vi "AudioTest.Pololu.Dual_Servo_Controller.vi"(11 "Module Config":T3={"Name"="DualServoCtrl", "Parent Q"=refnum, "Is Child?"=FALSE, "Index"=0, "Dirs"={"Root"=path "", "Config"=path "C:/ATE/Config", "Logs"=path "C:/ATE/Logs", "Reports"=path "C:/ATE/Reports", "App Data"=path "C:/ProgramData/MAIN"}, "Simulate"=FALSE, "SimCtrl"=refnum}) -> ()   [LabVIEW 2018]
uses:
  <vilib>/KATE/Module/Module Config.ctl
  <vilib>/KATE/Queues/Q.Element.ctl
  <vilib>/KATE/Module/Module.Working Dirs.ctl
  Common/Instruments/Servo Motors/Pololu/SubVIs/Pololu.Device Config.ctl
  Common/Instruments/Servo Motors/Pololu/SubVIs/Pololu.Device Range Config.ctl
  <vilib>/KATE/Module/Module.SW Version Info.ctl
  <vilib>/KATE/Module/Window/Window.Task, Action.ctl
  Common/Instruments/Servo Motors/Pololu/Dual Servo Manager Class/PololuCtrl.lvclass
  Common/Instruments/Servo Motors/Pololu/SubVIs/Pololu.Commands.ctl
  <vilib>/KATE/Config/Stored Controls/Class.SaveCtrls.lvclass
  <vilib>/KATE/Queues/Queue Utils.lvlib
  <vilib>/KATE/Module/Module Utils.lvlib
  <vilib>/KATE/Scheduler/Scheduler.lvlib
  <vilib>/KATE/Files/File Utils.lvlib
  <vilib>/KATE/Status/Status Utils.lvlib
  <vilib>/KATE/Event Log/Event Log.lvlib
panel:
  out "R Pos 3":dbl caption="Pos 0" format="%.1f"
  out "R Pos 2":dbl caption="Pos 1" format="%.1f"
  in  "Main Tab":enum32{"Operate", "Maint"}(tab)
  in  "Operate Tab":enum32{"Operate", "Config"}(tab)
  in  "Move All to 3":bool
  in  "R Step Dwn":bool
  in  "R Step Up":bool
  in  "L Step Dwn":bool
  in  "L Step Up":bool
  in  "Move All to 0":bool
  in  "Move All to 1":bool
  in  "R Go To Pos 0":bool
  in  "R Go To Pos 1":bool
  in  "Right Cmd Pos (Deg)":dbl(slide)=135.0 caption="Position (Deg)" max=270.0 scale=0.0..270.0 scale format="%.1f"
  out "R Pos 0":dbl caption="Pos 0" format="%.1f"
  out "R Pos 1":dbl caption="Pos 1" format="%.1f"
  in  "R Set Pos 0":bool
  in  "R Set Pos 1":bool
  in  "L Go To Pos 0":bool
  in  "L Go To Pos 1":bool
  in  "WaitTillDone":bool=TRUE caption="Wait Till Done"
  in  "Mov Timeout":dbl=5.0 caption="Timeout(s)"
  in  "Mov PosID":u8 caption="Position ID"
  in  "Mov Device":enum16{"Left", "Right", "All"}(ring)=enum."All" caption="Device"
  in  "Move Funct":bool
  in  "Left Cmd Pos (Deg)":dbl(slide)=135.0 caption="Position (Deg)" max=270.0 scale=0.0..270.0 scale format="%.1f"
  in  "Pos0 Invert":bool caption="Invert Scale"
  out "L Pos 0":dbl caption="Pos 0" format="%.1f"
  out "L Pos1":dbl caption="Pos 1" format="%.1f"
  in  "L Set Pos 0":bool
  in  "L Set Pos 1":bool
  out "Moving":bool
  in  "Pos1 Invert":bool caption="Invert Scale"
  out "Pos Cmd us":dbl[](array[numeric]) caption="Position Commands in us" format="%.1f"
  in  "0.25us/10ms/80ms":dbl=6.0
  in  "0.25us/10ms":dbl=100.0
  in  "Set Accel":bool
  in  "Set Speed":bool
  out "Read Errors":u16 max=270 format="%016b"
  in  "Get Errors":bool
  out "Error":errorcluster
  in  "Get Pos":bool
  out "Status Pos(Deg)":dbl[](array[numeric]) format="%.1f"
  out "Left Cmd Pos(us)":dbl
  out "Right Cmd Pos(us)":dbl
  in  "PID":string="0089"
  in  "VID":string="1FFB"
  out "Device Config":T1[](array[typedef])
  out "Config Dir":path
  out "CLI Args":string[](array[string])
  out "Connected":bool
  in  "Connect":bool
  in  "Disconnect":bool
  out "Port":string
  out "Error Status":string
  in  "R Set Upper Stop":bool
  out "R Upper Stop":dbl format="%.1f"
  in  "L Set Upper Stop":bool
  out "L Upper Stop":dbl format="%.1f"
  in  "L Set Lower Stop":bool
  out "L Lower Stop":dbl format="%.1f"
  in  "R Set Lower Stop":bool
  out "R Lower Stop":dbl format="%.1f"
  in  "Ignore Stops":bool=TRUE
  in  "Reset Stops":bool
  # "Detailed Function"
  # "Dual Servo Controller"
  # "Summary Functions"
  # "LEFT"
  # "RIGHT"
  # "Move(1,All)"
  # "Move(0,All)"
  # "Move(3,All)"
  # "Move(PosID,[Devices, Wait,Timeout])"
  # "Baby Step"
  # "Baby Step"
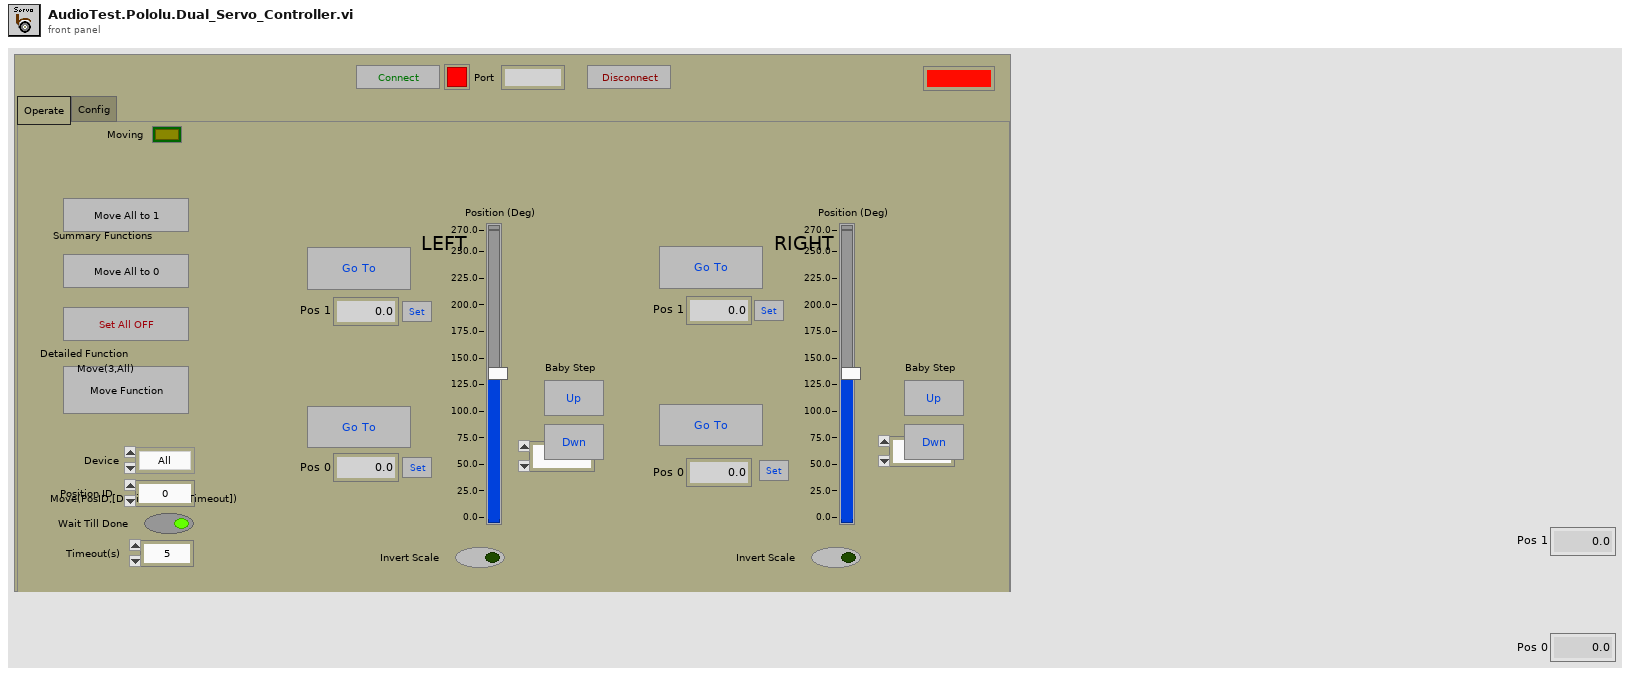
[diagram p1: front panel]
types:
  T1 = typedef "Pololu.Device Config.ctl" = cluster{"Chan":u8, "Accel":u16, "Speed":u16, "Positions":dbl[], "Range Info":T2}
  T2 = typedef "Pololu.Device Range Config.ctl" = cluster{"Min us":dbl, "Max us":dbl, "Min deg":dbl, "Max deg":dbl, "LStopDeg":dbl, "UStopDeg":dbl}
  T3 = typedef "KATE_Lib.lvlib/Module Utils.lvlib/Module Config.ctl" = cluster{"Name":string, "Parent Q":refnum<queue>, "Is Child?":bool, "Index":i32, "Dirs":T4, "Simulate":bool, "SimCtrl":refnum<vi>}
  T4 = typedef "KATE_Lib.lvlib/Module Utils.lvlib/Module.Working Dirs.ctl" = cluster{"Root":path, "Config":path, "Logs":path, "Reports":path, "App Data":path}
  T5 = typedef "KATE_Lib.lvlib/Module Utils.lvlib/Module.SW Version Info.ctl" = cluster{"AppName":string, "Company":string, "Version":string, "Description":string, "PN":string}
  T6 = typedef "KATE_Lib.lvlib/Module Utils.lvlib/Module Sys Info.ctl" = cluster{"Main Q":refnum<queue>, "Exe":bool, "SW Rev":T5, "Self Ref":refnum<vi>, "Main Tab":refnum<vi>, "Pane":refnum<vi>, "Stop":cluster{"Ref":refnum<event-registration>, "Event":refnum<user-event>}, "Cfg":T3, "Services":cluster{"Name":string, "vi ref":refnum<vi>}[], "Menu Ref":refnum<k9>, "CtrlStates":refnum<class "Class.SaveCtrls.lvclass">, "Docs":cluster{"Tags":string[], "Paths":path[]}, "Log":refnum<class "Event Notification.lvclass">, "Test Controls":refnum<vi>[], "Child Modules":cluster{"Name":string, "vi ref":refnum<vi>}[], "SW Items":string[][], "AppData":refnum<class "Class.AppData.lvclass">, "Subscriptions":refnum<class "Subscription.lvclass">}
  T7 = enum32{"Invalid", "Standard", "Closed", "Hidden", "Minimized", "Maximized"}
  T8 = enum16{"Left Upper Stop", "Left Lower Stop", "Left Pos 0", "Left Pos 1", "Right Upper Stop", "Right Lower Stop", "Right Pos 0", "Right Pos 1"}
  T9 = typedef "Pololu.Commands.ctl" = enum16{"Set Pos", "Set Speed", "Set Accel", "Get Pos", "Get Mov Status", "Get Errors"}
  T10 = cluster{"Active":bool, "Test":string, "Args":string[]}
  T11 = cluster{"Pololu":refnum<class "PololuCtrl.lvclass">, "CLI":cluster{"Active":bool, "Test":string, "Args":string[]}}
  T12 = cluster{"Device":enum16{"Left", "Right", "All"}, "PosID":u8, "Wait":bool, "Timeout":dbl}
  T13 = typedef "KATE_Lib.lvlib/Module Utils.lvlib/Window.Task, Action.ctl" = enum16{"Resize()", "Show Panel(Bool)", "Show Scroll Bars(Bool)", "Dock to SubPanel(SubPanel Ref)", "Undock from SubPanel()", "Return to SubPanel()", "Go To Maint Tab()", "Show Maint Tab(Bool)", "Open Block Diagram()"}
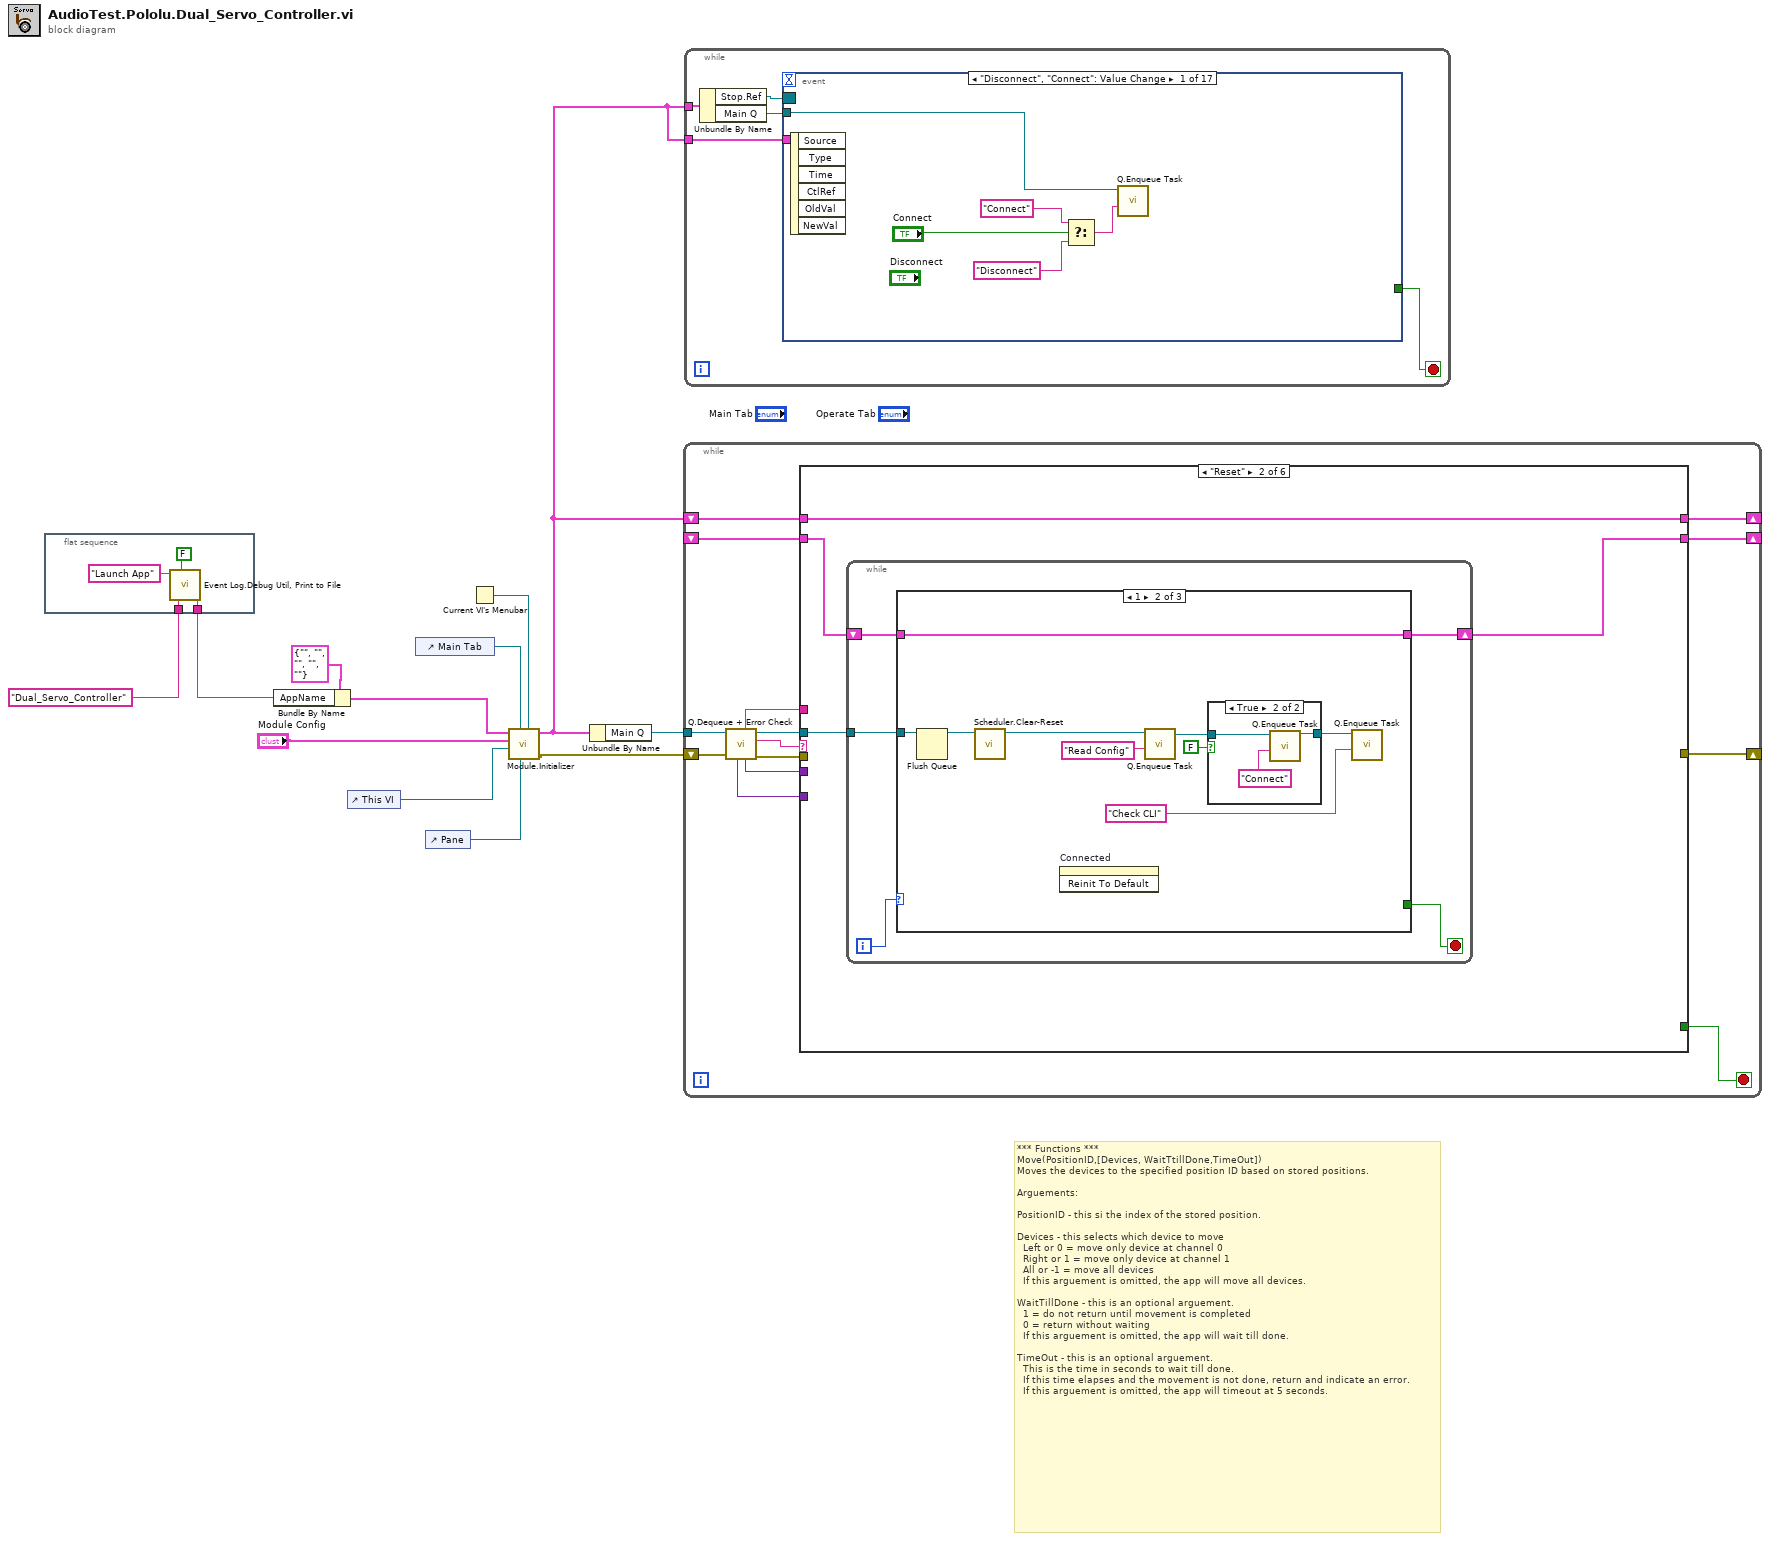
[diagram p0: block diagram]
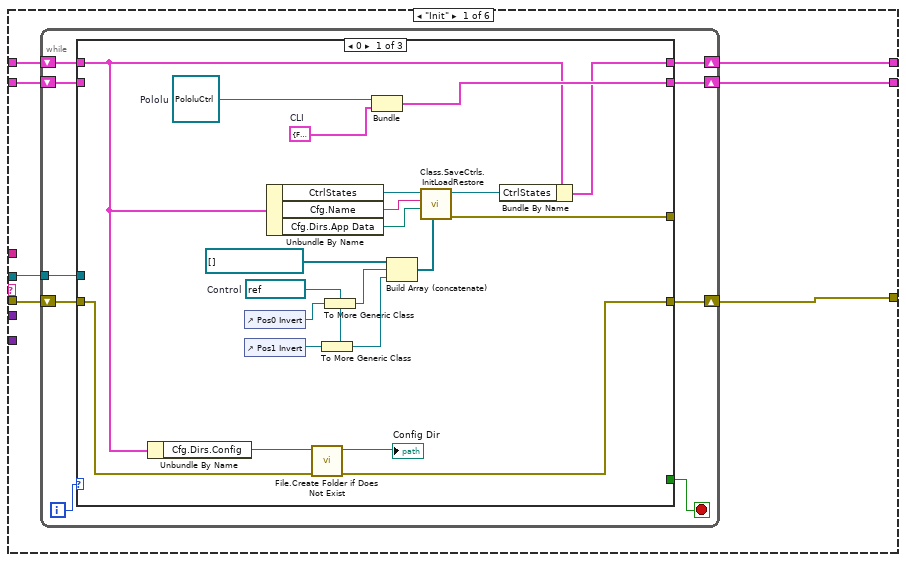
[diagram p2: hidden frame]
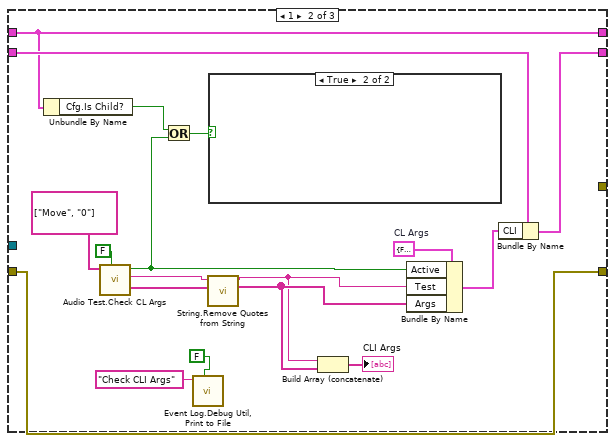
[diagram p3: hidden frame]
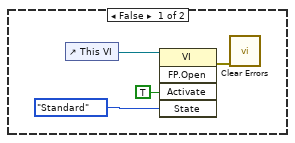
[diagram p4: hidden frame]
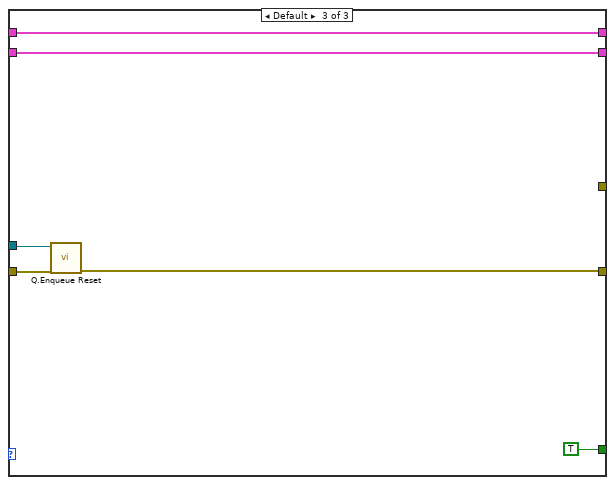
[diagram p5: hidden frame]
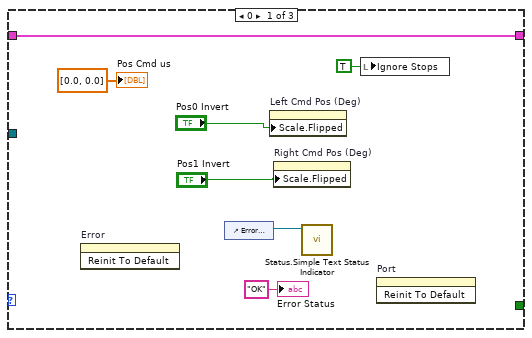
[diagram p6: hidden frame]
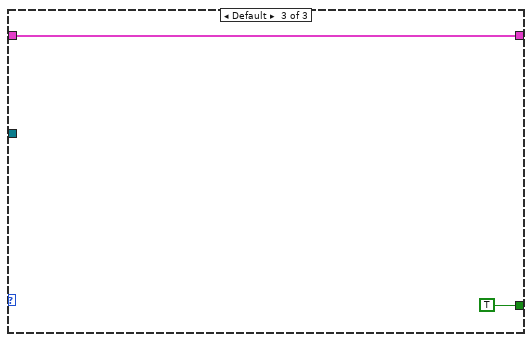
[diagram p8: hidden frame]
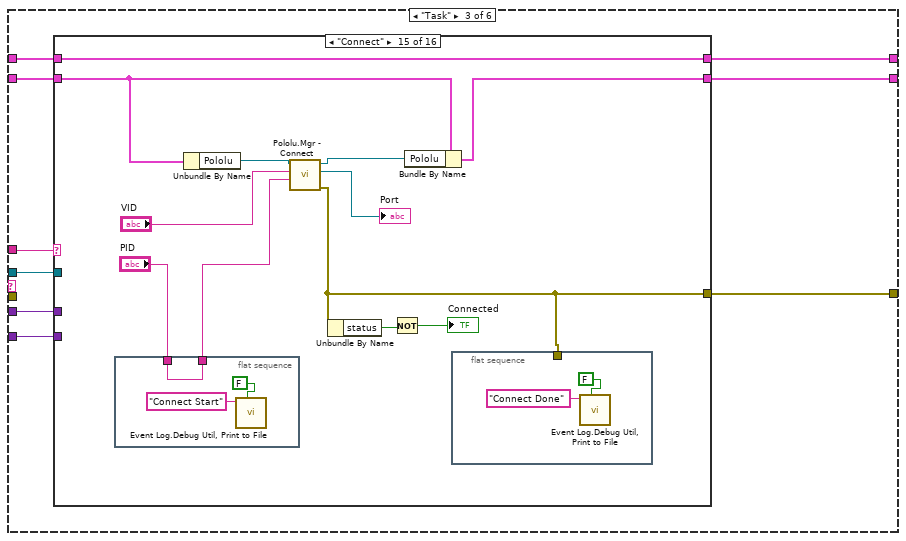
[diagram p9: hidden frame]
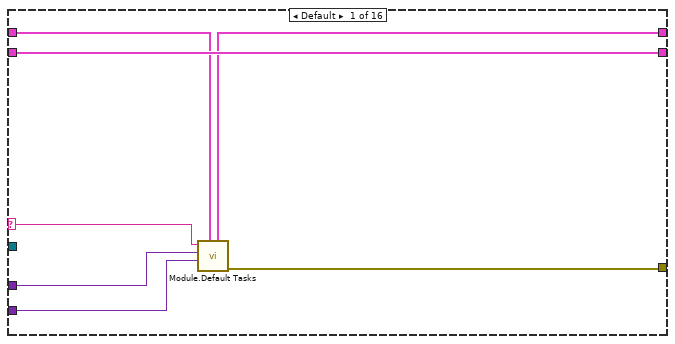
[diagram p10: hidden frame]
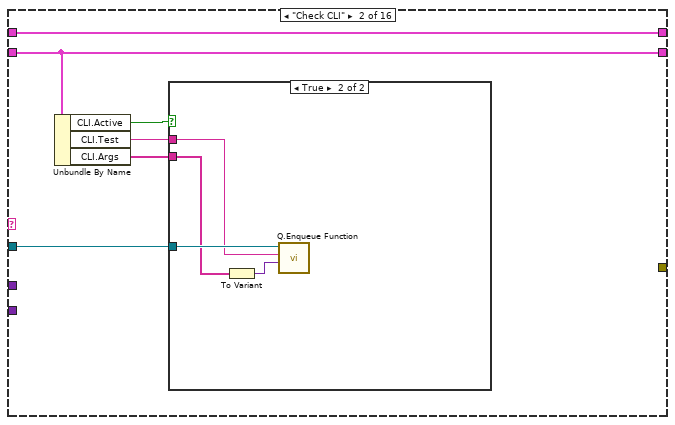
[diagram p11: hidden frame]
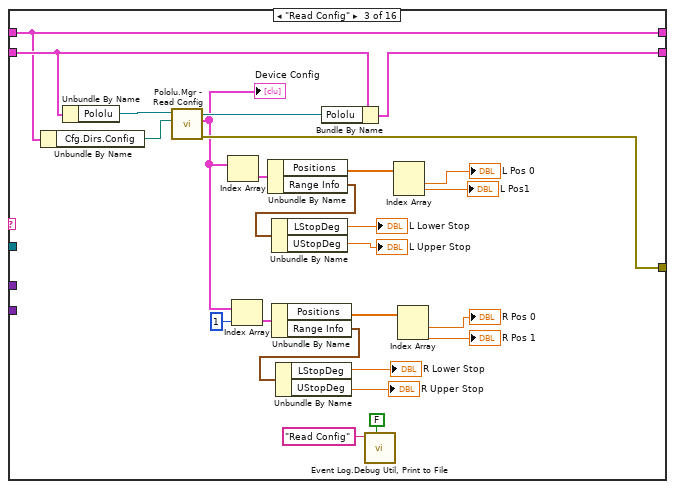
[diagram p13: hidden frame]
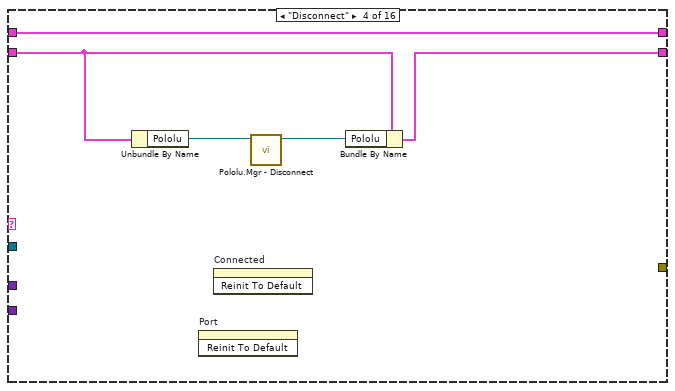
[diagram p14: hidden frame]
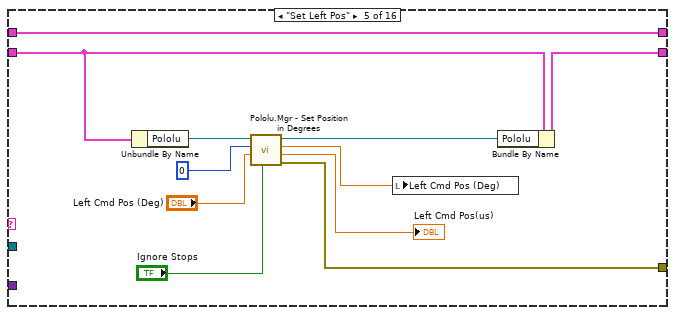
[diagram p15: hidden frame]
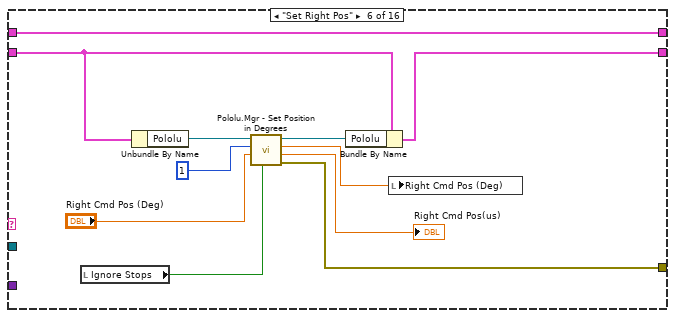
[diagram p16: hidden frame]
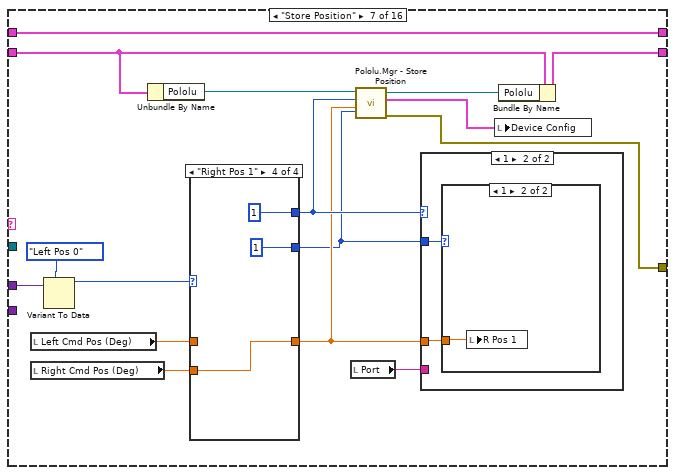
[diagram p17: hidden frame]
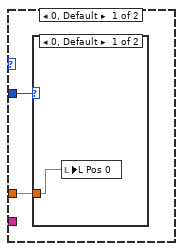
[diagram p18: hidden frame]
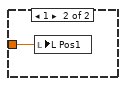
[diagram p19: hidden frame]
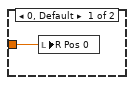
[diagram p20: hidden frame]
diagram:
  # "*** Functions ***\nMove(PositionID,[Devices, WaitTtillDone,TimeOut])\nMoves the devices to the specified position ID based on stored positions.\n\nArguements:\n\nPositionID - this si the index of the stored position.\n\nDevices - this selects which device to move\n  Left or 0 = move only device at channel 0\n  Right or 1 = move only device at channel 1\n  All or -1 = move all devices\n  If this arguement is omitted, the app will move all devices.\n\nWaitTillDone - this is an optional arguement.\n  1 = do not return until movement is completed\n  0 = return without waiting\n  If this arguement is omitted, the app will wait till done.\n\nTimeOut - this is an optional arguement.\n  This is the time in seconds to wait till done.\n  If this time elapses and the movement is not done, return and indicate an error.\n  If this arguement is omitted, the app will timeout at 5 seconds."
  n1 = flat-sequence {
    tunnel: [w14] -> w2
    tunnel: "Dual_Servo_Controller" ("AppName") -> [w14]
    frame #0 {
      n2 = call <vilib>:"Event Log.Debug Util, Print to File.vi"("Enable"=FALSE, "Message"="Launch App") -> ()  [unwired: 10 in]
    }
  }
  n3 = Bundle By Name(cluster=T5 {"AppName"="", "Company"="", "Version"="", "Description"="", "PN"=""} ("SW Rev"), "AppName"=w2) -> (w5:T5)
  n4 = control-ref of="This VI"() -> (w10:refnum<vi>)
  n5 = control-ref of="Main Tab"() -> (w8:refnum<vi>)
  n6 = control-ref of="Pane"() -> (w7:refnum<vi>)
  n7 = Current VI's Menubar() -> (w9:refnum<k9>)
  n8 = call <vilib>:"Module.Initializer.vi"("Menu Ref"=w9, "Pane"=w7, "Main Tab"=w8, "Self Ref"=w10, "Module Config"="Module Config", "SW Rev"=w5) -> ("error out"=w12:errorcluster, "Sys"=w3:T6)  [unwired: 4 in]
  n9 = Unbundle By Name(w3) -> ("Main Q"=w11:refnum<queue>)
  n10 = while {
    tunnel: w11 -> [w29]
    shift-right: [w20] -> _
    shift-left: w12 -> [w28]
    shift-right: [w18] -> _
    shift-left: _ -> [w22]
    shift-right: [w16] -> _
    shift-left: w3 -> [w17]
    stop <- w19 stop-if-true
    n11 = call <vilib>:"Q.Dequeue + Error Check.vi"("Error In"=w28, "Q In"=w29) -> ("error out"=w21:errorcluster, "Cmd"=w27:string, "Q Out"=w26:refnum<queue>, "Data1"=w24:variant, "Sub"=w25:string, "Data2"=w23:variant)  [unwired: 4 in]
    n12 = case shown="\"Reset\"" w27 {
      tunnel: w26 -> [w35 w98 w128 w390 _ _]
      tunnel: w25 -> [_ _ w134 w391 w565 _]
      tunnel: w24 -> [_ _ w127 w389 w571 _]
      tunnel: w23 -> [_ _ w126 w388 _ _]
      tunnel: w22 -> [w30 w95 w133 w393 w569 w589]
      tunnel: w21 -> [w32 _ _ w384 w572 _]
      tunnel: [w31 _ w131 _ errorcluster {"status"=FALSE, "code"=0, "source"=""} ("error") _] -> w20
      tunnel: [_ _ _ _ _ TRUE] -> w19
      tunnel: [w36 w96 w132 w392 w569 w589] -> w18
      tunnel: w17 -> [w33 w97 w130 w394 w567 w588]
      tunnel: [w34 w97 w129 w394 w567 w588] -> w16
      frame "Init" {
        n13 = while {
          tunnel: w35 -> [w44]
          shift-right: [w43] -> w34
          shift-left: w33 -> [w42]
          shift-right: [w39] -> w31
          shift-left: w32 -> [w37]
          shift-right: [w45] -> w36
          shift-left: w30 -> [w38]
          i -> [w41]
          stop <- w40 stop-if-true
          n14 = case shown="0" w41 {
            tunnel: [w65 w78 w92] -> w45
            tunnel: w44 -> [_ _ w91]
            tunnel: [w62 w76 w89] -> w39
            tunnel: [w57 w74 w93] -> w43
            tunnel: w42 -> [w56 w74 w93]
            tunnel: [_ _ TRUE] -> w40
            tunnel: w38 -> [_ w75 w92]
            tunnel: w37 -> [w47 w76 w90]
            tunnel: [w46 _ _] -> _
            frame 0 {
              w48 = T10 {"Active"=FALSE, "Test"="", "Args"=[]}  # CLI
              w51 = refnum<vi> refnum  # Control
              w66 = refnum<class "PololuCtrl.lvclass"> refnum  # Pololu
              n15 = Unbundle By Name(w56) -> ("Cfg.Dirs.Config"=w64:path)
              n16 = control-ref of="Pos0 Invert"() -> (w52:refnum<vi>)
              n17 = control-ref of="Pos1 Invert"() -> (w50:refnum<vi>)
              n18 = Unbundle By Name(w56) -> ("CtrlStates"=w59:refnum<class "Class.SaveCtrls.lvclass">, "Cfg.Name"=w61:string, "Cfg.Dirs.App Data"=w60:path)
              n19 = call <vilib>:"File.Create Folder if Does Not Exist.vi"("error in"=w47, "Path"=w64) -> ("error out"=w62:errorcluster, "Dup Path"=→"Config Dir":path)  [unwired: 7 in, 1 out]
              n20 = To More Generic Class(target class=w51, reference=w50) -> (generic class reference=w49:refnum<vi>)
              n21 = To More Generic Class(target class=w51, reference=w52) -> (generic class reference=w53:refnum<vi>)
              n22 = Bundle("Pololu"=w66, "CLI"=w48) -> (w65:T11)  [unwired: 1 in]
              n23 = Build Array (concatenate)(refnum<vi>[] [], w53, w49) -> (w54:refnum<vi>[])
              n24 = call-dynamic "Class.SaveCtrls.InitLoadRestore.vi"("Ctrl Array"=w54, "Module Data Dir"=w60, "Module Name"=w61, "CtrlStates In"=w59) -> ("error out"=w46:errorcluster, "CtrlStates"=w58:refnum<class "Class.SaveCtrls.lvclass">)  [unwired: 6 in]
              n25 = Bundle By Name(cluster=w56, "CtrlStates"=w58) -> (w57:T6)
            }
            frame 1 {
              w79 = T10 {"Active"=FALSE, "Test"="", "Args"=[]}  # CL Args
              n26 = Unbundle By Name(w74) -> ("Cfg.Is Child?"=w72:bool)
              n27 = call "Audio Test.Check CL Args.vi"("Simulate"=FALSE, "Sim CL Args"=string[] ["Move", "0"]) -> ("Args"=w80:string[], "Action"=w81:string, "CmdLine"=w71:bool)  [unwired: 7 in]
              n28 = Or(x=w72, y=w71) -> (x .or. y?=w73:bool)
              n29 = call <vilib>:"Event Log.Debug Util, Print to File.vi"("Enable"=FALSE, "Message"="Check CLI Args") -> ()  [unwired: 10 in]
              n30 = call "String.Remove Quotes from String.vi"("1D String In"=w80, "String In"=w81) -> ("1D String without Quotes"=w84:string[], "String without Quotes"=w83:string)  [unwired: 7 in, 1 out]
              n31 = case shown="True" w73 {
                frame False {
                  n32 = control-ref of="This VI"() -> (w87:refnum<vi>)
                  n33 = invoke class="VI" method="FP.Open"(reference=w87, "Activate"=TRUE ("Activate?"), "State"=T7."Standard") -> (error out=w88:errorcluster)  [unwired: 2 in, 4 out]
                  n34 = call <vilib>:"Clear Errors.vi"("error in (no error)"=w88) -> ()  [unwired: 5 in, 2 out]
                }
                frame True {
                }
              }
              n35 = Build Array (concatenate)(w83, w84) -> (→"CLI Args":string[])
              n36 = Bundle By Name(cluster=w79, "Active"=w71, "Test"=w83, "Args"=w84) -> (w77:T10)
              n37 = Bundle By Name(cluster=w75, "CLI"=w77) -> (w78:T11)
            }
            frame Default {
              n38 = call <vilib>:"Q.Enqueue Reset.vi"("Error In"=w90, "Q In"=w91) -> ("error out"=w89:errorcluster)  [unwired: 8 in, 1 out]
            }
          }
        }
      }
      frame "Reset" {
        n39 = while {
          tunnel: w98 -> [w103]
          shift-right: [w100] -> w96
          shift-left: w95 -> [w101]
          i -> [w102]
          stop <- w99 stop-if-true
          n40 = case shown="1" w102 {
            tunnel: w103 -> [_ w116 _]
            tunnel: w101 -> [w110 w117 w125]
            tunnel: [w110 w117 w125] -> w100
            tunnel: [_ _ TRUE] -> w99
            frame 0 {
              n41 = invoke on="Error" class="Clust (strict)" method="Reinit To Default"() -> ()  [unwired: 3 in, 3 out]
              n42 = control-ref of="Error Status"() -> (w108:refnum<vi>)
              n43 = property on="Left Cmd Pos (Deg)" class="Slide (strict)"("Scale.Flipped"="Pos0 Invert") -> ()  [unwired: 2 in, 2 out]
              n44 = property on="Right Cmd Pos (Deg)" class="Slide (strict)"("Scale.Flipped"="Pos1 Invert") -> ()  [unwired: 2 in, 2 out]
              n45 = call <vilib>:"Status.Simple Text Status Indicator.vi"("Status TextBox"=w108) -> ()  [unwired: 10 in, 1 out]
              n46 = local write "Ignore Stops"(TRUE ("Ignore Stops")) -> ()
              n47 = invoke on="Port" class="Str" method="Reinit To Default"() -> ()  [unwired: 3 in, 3 out]
              "Error Status" <- "OK" ("Error Status")
              "Pos Cmd us" <- dbl[] [0.0, 0.0] ("Pos Cmd us")
            }
            frame 1 {
              n48 = Flush Queue(queue=w116) -> (queue out=w115:refnum<queue>)  [unwired: 1 in, 2 out]
              n49 = call <vilib>:"Scheduler.Clear-Reset.vi"("Q In"=w115) -> ("Q Out"=w114:refnum<queue>)  [unwired: 9 in, 1 out]
              n50 = invoke on="Connected" class="Bool (strict)" method="Reinit To Default"() -> ()  [unwired: 3 in, 3 out]
              n51 = call <vilib>:"Q.Enqueue Task.vi"("Task Name"="Read Config", "Q In"=w114) -> ("Q Out"=w118:refnum<queue>)  [unwired: 8 in, 1 out]
              n52 = case shown="True" FALSE {
                tunnel: w118 -> [w120 w122]
                tunnel: [w120 w121] -> w113
                frame False {
                }
                frame True {
                  n53 = call <vilib>:"Q.Enqueue Task.vi"("Task Name"="Connect", "Q In"=w122) -> ("Q Out"=w121:refnum<queue>)  [unwired: 8 in, 1 out]
                }
              }
              n54 = call <vilib>:"Q.Enqueue Task.vi"("Task Name"="Check CLI", "Q In"=w113) -> ()  [unwired: 8 in, 2 out]
            }
            frame Default {
            }
          }
        }
      }
      frame "Task" {
        n55 = case shown="\"Connect\"" w134 {
          selector: w134 -> [w140 _ _ _ _ _ _ _ _ _ _ _ w328 _ _ _]
          tunnel: w133 -> [w141 w146 w174 w181 w192 w203 w215 w250 w283 w305 w313 w321 w331 w351 w375 w382]
          tunnel: [w141 w146 w175 w180 w191 w202 w216 w251 w284 w304 w312 w320 w330 w352 w374 w382] -> w132
          tunnel: [w135 _ w172 _ w188 w199 w205 w240 w276 w301 w309 w316 w322 w337 w364 _] -> w131
          tunnel: w130 -> [w138 w147 w171 w177 w187 w198 w219 w254 w287 w300 w311 w314 w329 w353 w367 w381]
          tunnel: [w139 w147 w171 w177 w187 w198 w219 w254 w287 w300 w311 w314 w329 w353 w367 w381] -> w129
          tunnel: w128 -> [_ w144 _ _ _ _ _ _ _ _ _ _ w327 _ _ _]
          tunnel: w127 -> [w137 _ _ _ _ _ w212 w247 w281 _ _ _ _ _ _ _]
          tunnel: w126 -> [w136 _ _ _ _ _ _ _ _ _ _ _ _ _ _ _]
          frame Default {
            n56 = call <vilib>:"Module.Default Tasks.vi"("Sys"=w138, "Data2"=w136, "Data1"=w137, "Sub"=w140) -> ("error out"=w135:errorcluster, "Sys Out"=w139:T6)  [unwired: 6 in]
          }
          frame "Check CLI" {
            n57 = Unbundle By Name(w146) -> ("CLI.Active"=w145:bool, "CLI.Test"=w143:string, "CLI.Args"=w142:string[])
            n58 = case shown="True" w145 {
              tunnel: w144 -> [_ w151]
              tunnel: w143 -> [_ w150]
              tunnel: w142 -> [_ w148]
              frame False {
              }
              frame True {
                n59 = To Variant(anything=w148) -> (Variant=w149:variant)
                n60 = call <vilib>:"Q.Enqueue Function.vi"("Data1"=w149, "Task Name"=w150, "Q In"=w151) -> ()  [unwired: 6 in, 3 out]
              }
            }
          }
          frame "Read Config" {
            n61 = Unbundle By Name(w171) -> ("Cfg.Dirs.Config"=w170:path)
            n62 = Unbundle By Name(w174) -> ("Pololu"=w176:refnum<class "PololuCtrl.lvclass">)
            n63 = call "Pololu.Mgr - Read Config.vi"("Config Folder"=w170, "PololuCtrl in"=w176) -> ("error out"=w172:errorcluster, "Devices"=w163:T1[], "PololuCtrl out"=w173:refnum<class "PololuCtrl.lvclass">)  [unwired: 7 in]
            "Device Config" <- w163
            n64 = Index Array(array=w163) -> (element=w169:T1)  [unwired: 1 in]
            n65 = Index Array(array=w163, index=1) -> (element=w164:T1)
            n66 = Unbundle By Name(w169) -> ("Positions"=w168:dbl[], "Range Info"=w167:T2)
            n67 = Unbundle By Name(w167) -> ("LStopDeg"=→"L Lower Stop":dbl, "UStopDeg"=→"L Upper Stop":dbl)
            n68 = Unbundle By Name(w164) -> ("Positions"=w165:dbl[], "Range Info"=w166:T2)
            n69 = Unbundle By Name(w166) -> ("LStopDeg"=→"R Lower Stop":dbl, "UStopDeg"=→"R Upper Stop":dbl)
            n70 = Bundle By Name(cluster=w174, "Pololu"=w173) -> (w175:T11)
            n71 = call <vilib>:"Event Log.Debug Util, Print to File.vi"("Enable"=FALSE, "Message"="Read Config") -> ()  [unwired: 10 in]
            n72 = Index Array(array=w168) -> (element #1=→"L Pos 0":dbl, element #2=→"L Pos1":dbl)  [unwired: 2 in]
            n73 = Index Array(array=w165) -> (element #1=→"R Pos 0":dbl, element #2=→"R Pos 1":dbl)  [unwired: 2 in]
          }
          frame "Disconnect" {
            n74 = Unbundle By Name(w181) -> ("Pololu"=w179:refnum<class "PololuCtrl.lvclass">)
            n75 = invoke on="Port" class="Str" method="Reinit To Default"() -> ()  [unwired: 3 in, 3 out]
            n76 = invoke on="Connected" class="Bool (strict)" method="Reinit To Default"() -> ()  [unwired: 3 in, 3 out]
            n77 = call "Pololu.Mgr - Disconnect.vi"("PololuCtrl in"=w179) -> ("PololuCtrl out"=w178:refnum<class "PololuCtrl.lvclass">)  [unwired: 9 in, 1 out]
            n78 = Bundle By Name(cluster=w181, "Pololu"=w178) -> (w180:T11)
          }
          frame "Set Left Pos" {
            n79 = Unbundle By Name(w192) -> ("Pololu"=w190:refnum<class "PololuCtrl.lvclass">)
            n80 = call "Pololu.Mgr - Set Position in Degrees.vi"("Ignore Stops"="Ignore Stops", "Pos(Deg)"="Left Cmd Pos (Deg)", "Channel"=u8 0, "PololuCtrl in"=w190) -> ("error out"=w188:errorcluster, "Actual Pos(us)"=→"Left Cmd Pos(us)":dbl, "Actual Pos(Deg)"=w186:dbl, "PololuCtrl out"=w189:refnum<class "PololuCtrl.lvclass">)  [unwired: 4 in]
            n81 = local write "Left Cmd Pos (Deg)"(w186) -> ()
            n82 = Bundle By Name(cluster=w192, "Pololu"=w189) -> (w191:T11)
          }
          frame "Set Right Pos" {
            n83 = local read "Ignore Stops"() -> (w193:bool)
            n84 = Unbundle By Name(w203) -> ("Pololu"=w201:refnum<class "PololuCtrl.lvclass">)
            n85 = call "Pololu.Mgr - Set Position in Degrees.vi"("Ignore Stops"=w193, "Pos(Deg)"="Right Cmd Pos (Deg)", "Channel"=u8 1, "PololuCtrl in"=w201) -> ("error out"=w199:errorcluster, "Actual Pos(us)"=→"Right Cmd Pos(us)":dbl, "Actual Pos(Deg)"=w197:dbl, "PololuCtrl out"=w200:refnum<class "PololuCtrl.lvclass">)  [unwired: 4 in]
            n86 = Bundle By Name(cluster=w203, "Pololu"=w200) -> (w202:T11)
            n87 = local write "Right Cmd Pos (Deg)"(w197) -> ()
          }
          frame "Store Position" {
            n88 = local read "Left Cmd Pos (Deg)"() -> (w210:dbl)
            n89 = local read "Right Cmd Pos (Deg)"() -> (w209:dbl)
            n90 = Variant To Data(type=T8."Left Pos 0", Variant=w212) -> (data=w211:T8)  [unwired: 1 in, 1 out]
            n91 = Unbundle By Name(w215) -> ("Pololu"=w218:refnum<class "PololuCtrl.lvclass">)
            n92 = case shown="\"Right Pos 1\"" w211 {
              tunnel: w210 -> [w229 w232 _ _]
              tunnel: w209 -> [_ _ w234 w237]
              tunnel: [u8 0 ("Channel") u8 0 ("Channel") u8 1 ("Channel") u8 1 ("Channel")] -> w208
              tunnel: [w229 w232 w234 w237] -> w207
              tunnel: [0 ("Index") 1 ("Index") 0 ("Index") 1 ("Index")] -> w206
              frame "Left Pos 0", Default {
              }
              frame "Left Pos 1" {
              }
              frame "Right Pos 0" {
              }
              frame "Right Pos 1" {
              }
            }
            n93 = local read "Port"() -> (w204:string)
            n94 = call "Pololu.Mgr - Store Position.vi"("Index"=w206, "Pos(Deg)"=w207, "Channel"=w208, "PololuCtrl in"=w218) -> ("error out"=w205:errorcluster, "Device Config"=w214:T1[], "PololuCtrl out"=w217:refnum<class "PololuCtrl.lvclass">)  [unwired: 5 in]
            n95 = case shown="1" w208 {
              tunnel: w207 -> [w220 w225]
              tunnel: w206 -> [w221 w224]
              tunnel: w204 -> [_ _]
              frame 0, Default {
                n96 = case shown="0, Default" w221 {
                  tunnel: w220 -> [w222 w223]
                  frame 0, Default {
                    n97 = local write "L Pos 0"(w222) -> ()
                  }
                  frame 1 {
                    n98 = local write "L Pos1"(w223) -> ()
                  }
                }
              }
              frame 1 {
                n99 = case shown="1" w224 {
                  tunnel: w225 -> [w226 w227]
                  frame 0, Default {
                    n100 = local write "R Pos 0"(w226) -> ()
                  }
                  frame 1 {
                    n101 = local write "R Pos 1"(w227) -> ()
                  }
                }
              }
            }
            n102 = local write "Device Config"(w214) -> ()
            n103 = Bundle By Name(cluster=w215, "Pololu"=w217) -> (w216:T11)
          }
          frame "Store Stop Position" {
            n104 = local read "Left Cmd Pos (Deg)"() -> (w245:dbl)
            n105 = local read "Right Cmd Pos (Deg)"() -> (w244:dbl)
            n106 = Variant To Data(type=T8."Right Upper Stop", Variant=w247) -> (data=w246:T8)  [unwired: 1 in, 1 out]
            n107 = case shown="\"Left Upper Stop\", Default" w246 {
              tunnel: w245 -> [w264 w267 _ _]
              tunnel: w244 -> [_ _ w270 w273]
              tunnel: [u8 0 ("Channel") u8 0 ("Channel") u8 1 ("Channel") u8 1 ("Channel")] -> w243
              tunnel: [w264 w267 w270 w273] -> w241
              tunnel: [enum16{"Lower", "Upper"}."Upper" ("Type") enum16{"Lower", "Upper"}."Lower" ("Type") enum16{"Lower", "Upper"}."Upper" ("Type") enum16{"Lower", "Upper"}."Lower" ("Type")] -> w242
              frame "Left Upper Stop", Default {
              }
              frame "Left Lower Stop" {
              }
              frame "Right Upper Stop" {
              }
              frame "Right Lower Stop" {
              }
            }
            n108 = Unbundle By Name(w250) -> ("Pololu"=w253:refnum<class "PololuCtrl.lvclass">)
            n109 = call "Pololu.Mgr - Store Lower or Upper Stop Position.vi"("Type"=w242, "Pos(Deg)"=w241, "Channel"=w243, "PololuCtrl in"=w253) -> ("error out"=w240:errorcluster, "Device Config"=w249:T1[], "PololuCtrl out"=w252:refnum<class "PololuCtrl.lvclass">)  [unwired: 5 in]
            n110 = case shown="0, Default" w243 {
              tunnel: w241 -> [w255 w260]
              tunnel: w242 -> [w256 w259]
              frame 0, Default {
                n111 = case shown="\"Upper\"" w256 {
                  tunnel: w255 -> [w257 w258]
                  frame "Lower", Default {
                    n112 = local write "L Lower Stop"(w257) -> ()
                  }
                  frame "Upper" {
                    n113 = local write "L Upper Stop"(w258) -> ()
                  }
                }
              }
              frame 1 {
                n114 = case shown="\"Lower\", Default" w259 {
                  tunnel: w260 -> [w261 w262]
                  frame "Lower", Default {
                    n115 = local write "R Lower Stop"(w261) -> ()
                  }
                  frame "Upper" {
                    n116 = local write "R Upper Stop"(w262) -> ()
                  }
                }
              }
            }
            n117 = local write "Device Config"(w249) -> ()
            n118 = Bundle By Name(cluster=w250, "Pololu"=w252) -> (w251:T11)
          }
          frame "Go To Saved Pos" {
            n119 = Variant To Data(type=T8."Left Pos 0", Variant=w281) -> (data=w280:T8)  [unwired: 1 in, 1 out]
            n120 = case shown="\"Right Pos 1\"" w280 {
              tunnel: [u8 0 ("Channel") u8 0 ("Channel") u8 1 ("Channel") u8 1 ("Channel")] -> w278
              tunnel: [0 ("Index") 1 ("Index") 0 ("Index") 1 ("Index")] -> w279
              frame "Left Pos 0", Default {
              }
              frame "Left Pos 1" {
              }
              frame "Right Pos 0" {
              }
              frame "Right Pos 1" {
              }
            }
            n121 = Unbundle By Name(w283) -> ("Pololu"=w286:refnum<class "PololuCtrl.lvclass">)
            n122 = local read "Ignore Stops"() -> (w275:bool)
            n123 = call "Pololu.Mgr - Move to Saved Position.vi"("Ignore Stops"=w275, "Position Index"=w279, "Channel"=w278, "PololuCtrl in"=w286) -> ("error out"=w276:errorcluster, "Position(Deg)"=w277:dbl, "PololuCtrl out"=w285:refnum<class "PololuCtrl.lvclass">)  [unwired: 3 in, 2 out]
            n124 = case shown="1" w278 {
              tunnel: w277 -> [w288 w289]
              frame 0, Default {
                n125 = local write "Left Cmd Pos (Deg)"(w288) -> ()
              }
              frame 1 {
                n126 = local write "Right Cmd Pos (Deg)"(w289) -> ()
              }
            }
            n127 = Bundle By Name(cluster=w283, "Pololu"=w285) -> (w284:T11)
          }
          frame "Set Accel" {
            # "All"
            # "Speed is in 0.25us/10ms\nAccel is in  0.25us/10ms/80ms"
            n128 = Unbundle By Name(w305) -> ("Pololu"=w303:refnum<class "PololuCtrl.lvclass">)
            n129 = call "Pololu.Mgr - Set Acceleration.vi"("0.25us/10ms/80ms"="0.25us/10ms/80ms", "Channel(use -1 for All)"=-1, "PololuCtrl in"=w303) -> ("error out"=w301:errorcluster, "PololuCtrl out"=w302:refnum<class "PololuCtrl.lvclass">)  [unwired: 7 in]
            n130 = Bundle By Name(cluster=w305, "Pololu"=w302) -> (w304:T11)
          }
          frame "Set Speed" {
            # "Speed is in 0.25us/10ms\nAccel is in  0.25us/10ms/80ms"
            n131 = Unbundle By Name(w313) -> ("Pololu"=w307:refnum<class "PololuCtrl.lvclass">)
            n132 = call "Pololu.Mgr - Set Speed.vi"("0.25us/10ms"="0.25us/10ms", "Channel(use -1 for All)"=-1, "PololuCtrl in"=w307) -> ("error out"=w309:errorcluster, "PololuCtrl out"=w310:refnum<class "PololuCtrl.lvclass">)  [unwired: 7 in]
            n133 = Bundle By Name(cluster=w313, "Pololu"=w310) -> (w312:T11)
          }
          frame "Read Errors" {
            n134 = Unbundle By Name(w321) -> ("Pololu"=w319:refnum<class "PololuCtrl.lvclass">)
            n135 = call "Pololu.Mgr - Send Message to Pololu.vi"("Command"=Pololu.Commands."Get Errors", "PololuCtrl in"=w319) -> ("error out"=w316:errorcluster, "Response"=→"Read Errors":u16, "PololuCtrl out"=w318:refnum<class "PololuCtrl.lvclass">)  [unwired: 7 in]
            n136 = Bundle By Name(cluster=w321, "Pololu"=w318) -> (w320:T11)
          }
          frame "Get Status" {
            n137 = Unbundle By Name(w331) -> ("Pololu"=w326:refnum<class "PololuCtrl.lvclass">)
            n138 = call "Pololu.Mgr - Get Status.vi"("PololuCtrl in"=w326) -> ("error out"=w322:errorcluster, "Pos(Deg)"=→"Status Pos(Deg)":dbl[], "Moving"=w323:bool, "PololuCtrl out"=w325:refnum<class "PololuCtrl.lvclass">)  [unwired: 7 in]
            "Moving" <- w323
            n139 = Bundle By Name(cluster=w331, "Pololu"=w325) -> (w330:T11)
            n140 = case shown="True" w323 {
              tunnel: w327 -> [_ w335]
              tunnel: w328 -> [_ w333]
              tunnel: [_ w334] -> _
              frame False {
              }
              frame True {
                n141 = call <vilib>:"Scheduler.AddTask.vi"("Interval(s)"=0.2, "Task Name"=w333, "Sched Name"=w333, "Q In"=w335) -> ("Error Out"=w334:errorcluster)  [unwired: 6 in, 1 out]
              }
            }
          }
          frame "Reset Stop Positions" {
            n142 = local read "Pos1 Invert"() -> (w342:bool)
            n143 = local read "Pos0 Invert"() -> (w343:bool)
            n144 = Unbundle By Name(w351) -> ("Pololu"=w355:refnum<class "PololuCtrl.lvclass">)
            n145 = call "Pololu.Mgr - Get Device Config.vi"("PololuCtrl in"=w355) -> ("error out"=w336:errorcluster, "Device Config"=w348:T1[], "PololuCtrl out"=w354:refnum<class "PololuCtrl.lvclass">)  [unwired: 8 in]
            n146 = case shown="True" w343 {
              tunnel: [270.0 0.0] -> w338
              tunnel: [0.0 270.0] -> w339
              frame False {
              }
              frame True {
              }
            }
            n147 = case shown="True" w342 {
              tunnel: [270.0 0.0] -> w340
              tunnel: [0.0 270.0] -> w341
              frame False {
              }
              frame True {
              }
            }
            n148 = Index Array(array=w348) -> (element #1=w349:T1, element #2=w344:T1)  [unwired: 2 in]
            n149 = Bundle By Name(cluster=w349, "Range Info.UStopDeg"=w338, "Range Info.LStopDeg"=w339) -> (w347:T1)
            n150 = Bundle By Name(cluster=w344, "Range Info.UStopDeg"=w340, "Range Info.LStopDeg"=w341) -> (w346:T1)
            n151 = local write "L Lower Stop"(w339) -> ()
            n152 = local write "L Upper Stop"(w338) -> ()
            n153 = local write "R Upper Stop"(w340) -> ()
            n154 = local write "R Lower Stop"(w341) -> ()
            n155 = Build Array(w347, w346) -> (w345:T1[])
            n156 = call "Pololu.Mgr - Set Device Config.vi"("error in (no error)"=w336, "Device Config"=w345, "PololuCtrl in"=w354) -> ("error out"=w337:errorcluster, "PololuCtrl out"=w350:refnum<class "PololuCtrl.lvclass">)  [unwired: 7 in]
            n157 = Bundle By Name(cluster=w351, "Pololu"=w350) -> (w352:T11)
          }
          frame "Connect" {
            n158 = flat-sequence {
              tunnel: [w379] -> w365
              tunnel: "PID" -> [w379]
              frame #0 {
                n159 = call <vilib>:"Event Log.Debug Util, Print to File.vi"("Enable"=FALSE, "Message"="Connect Start") -> ()  [unwired: 10 in]
              }
            }
            n160 = Unbundle By Name(w375) -> ("Pololu"=w373:refnum<class "PololuCtrl.lvclass">)
            n161 = call "Pololu.Mgr - Connect.vi"("PID"=w365, "VID"="VID", "PololuCtrl in"=w373) -> ("error out"=w364:errorcluster, "Com Port"=→"Port":refnum<visa-resource-name>, "PololuCtrl out"=w372:refnum<class "PololuCtrl.lvclass">)  [unwired: 6 in]
            n162 = Unbundle By Name(w364) -> ("status"=w369:bool)
            n163 = Not(x=w369) -> (.not. x?=→"Connected":bool)
            n164 = Bundle By Name(cluster=w375, "Pololu"=w372) -> (w374:T11)
            n165 = flat-sequence {
              tunnel: w364 -> [_]
              frame #0 {
                n166 = call <vilib>:"Event Log.Debug Util, Print to File.vi"("Enable"=FALSE, "Message"="Connect Done") -> ()  [unwired: 10 in]
              }
            }
          }
          frame "Local RTN" {
            # "Do Nothing"
          }
        }
      }
      frame "Function" {
        n167 = case shown="\"Move\"" w391 {
          tunnel: w393 -> [w400 w407]
          tunnel: [w400 w406] -> w392
          tunnel: w390 -> [_ w401]
          tunnel: w389 -> [_ w408]
          tunnel: [variant _] -> w387
          tunnel: [TRUE ("Active") w405] -> w386
          tunnel: "Init" -> [_ w404]
          tunnel: w384 -> [_ w403]
          tunnel: [_ w402] -> w383
          frame Default {
          }
          frame "Move" {
            n168 = while {
              tunnel: w408 -> [w421]
              tunnel: [w410] -> w405
              shift-right: [w419] -> w406
              shift-left: w407 -> [w420]
              shift-right: [w417] -> _
              shift-left: w404 -> [w418]
              shift-right: [w413] -> w402
              shift-left: w403 -> [w414]
              shift-right: [w411] -> _
              shift-left: _ -> [w412]
              tunnel: w401 -> [w409]
              stop <- w415 stop-if-true
              n169 = case shown="\"Init\"" w418 {
                tunnel: w421 -> [w436 _ _ _ _]
                tunnel: w420 -> [w434 w441 w453 w528 w556]
                tunnel: [w434 w442 w454 w529 w556] -> w419
                tunnel: ["Connect" "Move" w460 "Done" "Done"] -> w416
                tunnel: [_ _ _ _ TRUE] -> w415
                tunnel: w414 -> [_ _ _ _ w558]
                tunnel: [_ w438 w450 w527 w558] -> w413
                tunnel: w412 -> [_ w449 w452 w532 w557]
                tunnel: [w429 w449 w452 w532 w557] -> w411
                tunnel: [_ _ _ _ w554] -> w410
                tunnel: w409 -> [_ _ _ _ w555]
                frame "Init" {
                  # "Move(PositionID,[Devices, WaitTtillDone,TimeOut])"
                  n170 = Variant To Data(type=string[] [], Variant=w436) -> (data=w431:string[], error out=w432:errorcluster)  [unwired: 1 in]
                  n171 = case shown="No Error" w432 {
                    tunnel: w431 -> [w437 _]
                    tunnel: [w437 _] -> w430
                    frame No Error {
                    }
                    frame Error {
                    }
                  }
                  n172 = call "Pololu.Dual Servo Parse Args for Funct Move.vi"("Args"=w430) -> ("Params"=w429:T12)  [unwired: 10 in]
                  n173 = Unbundle By Name(w429) -> ("Device"=w428:enum16{"Left", "Right", "All"}, "PosID"=w427:u8, "Wait"=w426:bool, "Timeout"=w425:dbl)
                  n174 = call <vilib>:"Event Log.Debug Util, Print to File.vi"("Enable"=FALSE, "Message"="Init Funct Move") -> ()  [unwired: 10 in]
                  n175 = local write "Mov PosID"(w427) -> ()
                  n176 = local write "WaitTillDone"(w426) -> ()
                  n177 = local write "Mov Timeout"(w425) -> ()
                  n178 = local write "Mov Device"(w428) -> ()
                  n179 = local write "Connected"(FALSE ("Connected")) -> ()
                }
                frame "Connect" {
                  n180 = Unbundle By Name(w441) -> ("Pololu"=w444:refnum<class "PololuCtrl.lvclass">)
                  n181 = local read "PID"() -> (w446:string)
                  n182 = local read "VID"() -> (w445:string)
                  n183 = call "Pololu.Mgr - Connect.vi"("PID"=w446, "VID"=w445, "PololuCtrl in"=w444) -> ("error out"=w438:errorcluster, "Com Port"=w447:refnum<visa-resource-name>, "PololuCtrl out"=w443:refnum<class "PololuCtrl.lvclass">)  [unwired: 6 in]
                  n184 = Unbundle By Name(w438) -> ("status"=w439:bool)
                  n185 = local write "Port"(w447) -> ()
                  n186 = Not(x=w439) -> (.not. x?=w440:bool)
                  n187 = Bundle By Name(cluster=w441, "Pololu"=w443) -> (w442:T11)
                  n188 = local write "Connected"(w440) -> ()
                }
                frame "Move" {
                  n189 = Unbundle By Name(w452) -> ("Device"=w456:enum16{"Left", "Right", "All"}, "PosID"=w455:u8)
                  n190 = flat-sequence {
                    tunnel: [TRUE] -> w451
                    frame #0 {
                      n191 = call <vilib>:"Event Log.Debug Util, Print to File.vi"("Enable"=FALSE, "Message"="Send Move Cmd to Servo") -> ()  [unwired: 10 in]
                    }
                  }
                  n192 = case shown="\"All\", Default" w456 {
                    tunnel: w455 -> [w467 w487 w507]
                    tunnel: w453 -> [w469 w489 w509]
                    tunnel: [w468 w488 w508] -> w454
                    tunnel: [w466 w486 w506] -> w450
                    tunnel: w451 -> [_ _ _]
                    frame "All", Default {
                      n193 = case shown="Default" w467 {
                        selector: w467 -> [w475 _]
                        tunnel: w469 -> [w480 w485]
                        tunnel: [w477 w482] -> w468
                        tunnel: [w471 w481] -> w466
                        frame Default {
                          n194 = Unbundle By Name(w480) -> ("Pololu"=w479:refnum<class "PololuCtrl.lvclass">)
                          n195 = To Long Integer(number=w475) -> (32bit integer=w476:i32)
                          n196 = call "Pololu.Mgr - Move All to Saved Positions.vi"("Ignore Stops"=TRUE, "Position Index"=w476, "PololuCtrl in"=w479) -> ("error out"=w471:errorcluster, "Positions"=w472:dbl[], "PololuCtrl out"=w478:refnum<class "PololuCtrl.lvclass">)  [unwired: 6 in]
                          n197 = Index Array(array=w472) -> (element #1=w474:dbl, element #2=w473:dbl)  [unwired: 2 in]
                          n198 = local write "Left Cmd Pos (Deg)"(w474) -> ()
                          n199 = local write "Right Cmd Pos (Deg)"(w473) -> ()
                          n200 = Bundle By Name(cluster=w480, "Pololu"=w478) -> (w477:T11)
                        }
                        frame 3 {
                          n201 = Unbundle By Name(w485) -> ("Pololu"=w484:refnum<class "PololuCtrl.lvclass">)
                          n202 = call "Pololu.Mgr - Set All to OFF.vi"("PololuCtrl in"=w484) -> ("error out"=w481:errorcluster, "PololuCtrl out"=w483:refnum<class "PololuCtrl.lvclass">)  [unwired: 9 in]
                          n203 = Bundle By Name(cluster=w485, "Pololu"=w483) -> (w482:T11)
                        }
                      }
                    }
                    frame "Right" {
                      n204 = case shown="Default" w487 {
                        selector: w487 -> [w494 _]
                        tunnel: w489 -> [w498 w504]
                        tunnel: [w497 w503] -> w488
                        tunnel: [w491 w500] -> w486
                        frame Default {
                          n205 = Unbundle By Name(w498) -> ("Pololu"=w495:refnum<class "PololuCtrl.lvclass">)
                          n206 = To Long Integer(number=w494) -> (32bit integer=w493:i32)
                          n207 = call "Pololu.Mgr - Move to Saved Position.vi"("Ignore Stops"=TRUE, "Position Index"=w493, "Channel"=u8 1, "PololuCtrl in"=w495) -> ("error out"=w491:errorcluster, "Position(Deg)"=w492:dbl, "PololuCtrl out"=w496:refnum<class "PololuCtrl.lvclass">)  [unwired: 3 in, 2 out]
                          n208 = local write "Right Cmd Pos (Deg)"(w492) -> ()
                          n209 = Bundle By Name(cluster=w498, "Pololu"=w496) -> (w497:T11)
                        }
                        frame 3 {
                          n210 = Unbundle By Name(w504) -> ("Pololu"=w501:refnum<class "PololuCtrl.lvclass">)
                          n211 = call "Pololu.Mgr - Set Channel OFF.vi"("Channel"=u8 1, "PololuCtrl in"=w501) -> ("error out"=w500:errorcluster, "PololuCtrl out"=w502:refnum<class "PololuCtrl.lvclass">)  [unwired: 8 in]
                          n212 = Bundle By Name(cluster=w504, "Pololu"=w502) -> (w503:T11)
                        }
                      }
                    }
                    frame "Left" {
                      n213 = case shown="Default" w507 {
                        selector: w507 -> [w514 _]
                        tunnel: w509 -> [w518 w524]
                        tunnel: [w517 w523] -> w508
                        tunnel: [w511 w520] -> w506
                        frame Default {
                          n214 = Unbundle By Name(w518) -> ("Pololu"=w515:refnum<class "PololuCtrl.lvclass">)
                          n215 = To Long Integer(number=w514) -> (32bit integer=w513:i32)
                          n216 = call "Pololu.Mgr - Move to Saved Position.vi"("Ignore Stops"=TRUE, "Position Index"=w513, "Channel"=u8 0, "PololuCtrl in"=w515) -> ("error out"=w511:errorcluster, "Position(Deg)"=w512:dbl, "PololuCtrl out"=w516:refnum<class "PololuCtrl.lvclass">)  [unwired: 3 in, 2 out]
                          n217 = local write "Left Cmd Pos (Deg)"(w512) -> ()
                          n218 = Bundle By Name(cluster=w518, "Pololu"=w516) -> (w517:T11)
                        }
                        frame 3 {
                          n219 = Unbundle By Name(w524) -> ("Pololu"=w521:refnum<class "PololuCtrl.lvclass">)
                          n220 = call "Pololu.Mgr - Set Channel OFF.vi"("Channel"=u8 0, "PololuCtrl in"=w521) -> ("error out"=w520:errorcluster, "PololuCtrl out"=w522:refnum<class "PololuCtrl.lvclass">)  [unwired: 8 in]
                          n221 = Bundle By Name(cluster=w524, "Pololu"=w522) -> (w523:T11)
                        }
                      }
                    }
                  }
                  n222 = flat-sequence {
                    tunnel: w450 -> [_]
                    frame #0 {
                      n223 = call <vilib>:"Event Log.Debug Util, Print to File.vi"("Enable"=FALSE, "Message"="Done with send Move Cmd to Servo") -> ()  [unwired: 10 in]
                    }
                  }
                  n224 = Unbundle By Name(w452) -> ("Wait"=w459:bool)
                  n225 = Select(t="Wait", s=w459, f="Done") -> (s? t:f=w460:string)
                }
                frame "Wait" {
                  n226 = Unbundle By Name(w532) -> ("Timeout"=w531:dbl)
                  n227 = Unbundle By Name(w528) -> ("Pololu"=w533:refnum<class "PololuCtrl.lvclass">)
                  n228 = flat-sequence {
                    tunnel: [TRUE] -> w526
                    frame #0 {
                      n229 = call <vilib>:"Event Log.Debug Util, Print to File.vi"("Enable"=FALSE, "Message"="Start Wait") -> ()  [unwired: 10 in]
                    }
                  }
                  n230 = call <vilib>:"High Resolution Relative Seconds.vi"() -> ("relative seconds"=w535:dbl)
                  n231 = while {
                    tunnel: w535 -> [w543]
                    shift-right: [w547] -> w530
                    shift-left: w533 -> [w548]
                    tunnel: w531 -> [w541]
                    tunnel: [w539] -> w527
                    tunnel: w526 -> [_]
                    stop <- w545 stop-if-true
                    # "Elapsed"
                    n232 = call <vilib>:"High Resolution Relative Seconds.vi"() -> ("relative seconds"=w544:dbl)
                    n233 = Subtract(x=w544, y=w543) -> (x-y=w542:dbl)
                    n234 = Greater?(x=w542, y=w541) -> (0:w540:bool)
                    n235 = call "Pololu.Mgr - Get Status.vi"("PololuCtrl in"=w548) -> ("error out"=w539:errorcluster, "Pos(Deg)"=w550:dbl[], "Moving"=w546:bool, "PololuCtrl out"=w547:refnum<class "PololuCtrl.lvclass">)  [unwired: 7 in]
                    n236 = local write "Status Pos(Deg)"(w550) -> ()
                    n237 = local write "Moving"(w546) -> ()
                    n238 = Compound Arithmetic op=OR(w539, invert w546, w540) -> (w545:bool)
                    n239 = Wait (ms)(milliseconds to wait=u32 200) -> ()  [unwired: 1 out]
                  }
                  n240 = Bundle By Name(cluster=w528, "Pololu"=w530) -> (w529:T11)
                }
                frame "Done", Default {
                  n241 = Unbundle By Name(w556) -> ("CLI.Active"=w554:bool)
                  n242 = case shown="True" w554 {
                    tunnel: w555 -> [_ w562]
                    frame False {
                    }
                    frame True {
                      n243 = call <vilib>:"Q.Enqueue Exit.vi"("Top of Q(T)"=TRUE, "Q In"=w562) -> ()  [unwired: 8 in, 2 out]
                    }
                  }
                  n244 = local write "Moving"(FALSE ("Moving")) -> ()
                  n245 = call <vilib>:"Event Log.Debug Util, Print to File.vi"("Enable"=FALSE, "Message"="Move Funct Done") -> ()  [unwired: 10 in]
                }
              }
              n246 = call "Error.Case Redirect on Error.vi"("error in"=w413, "Next Case"=w416) -> ("Next Case Out"=w417:string)  [unwired: 9 in]
            }
          }
        }
        n247 = case shown="False" w386 {
          tunnel: w388 -> [w397 _]
          tunnel: w387 -> [w396 _]
          tunnel: w383 -> [w395 _]
          frame False {
            n248 = call <vilib>:"Q.Return Function Data.vi"("error in"=w395, "Data2"=w397, "Ret Data"=w396) -> ()  [unwired: 8 in, 1 out]
          }
          frame True {
          }
        }
      }
      frame "Error", Default {
        n249 = Unbundle By Name(w567) -> ("Cfg.Parent Q"=w566:refnum<queue>)
        n250 = case shown="\"Error\"" w565 {
          tunnel: w572 -> [w577 _]
          tunnel: [w577 w579] -> w563
          tunnel: w571 -> [_ w580]
          frame Default {
          }
          frame "Error" {
            n251 = Variant To Data(type=errorcluster {"status"=FALSE, "code"=0, "source"=""} ("error"), Variant=w580) -> (data=w579:errorcluster)  [unwired: 1 in, 1 out]
          }
        }
        "Error" <- w563
        n252 = Not A Number/Path/Refnum?(number/path/refnum=w566) -> (NaN/Path/Refnum?=w568:bool)
        n253 = case shown="False" w568 {
          tunnel: w566 -> [w576 _]
          tunnel: w563 -> [w573 _]
          frame False {
            w575 = "Error" ("Cmd")
            n254 = To Variant(anything=w573) -> (Variant=w574:variant)
            n255 = call <vilib>:"Q.Enqueue Item.vi"("Data1"=w574, "Sub"=w575, "Cmd"=w575, "Q In"=w576) -> ()  [unwired: 6 in, 2 out]
          }
          frame True {
          }
        }
        n256 = control-ref of="Error Status"() -> (w564:refnum<vi>)
        n257 = call <vilib>:"Status.Simple Text Status Indicator.vi"("error in"=w563, "Status TextBox"=w564) -> ()  [unwired: 9 in, 1 out]
      }
      frame "Exit" {
        n258 = Unbundle By Name(w589) -> ("Pololu"=w591:refnum<class "PololuCtrl.lvclass">)
        n259 = Unbundle By Name(w588) -> ("Exe"=w583:bool, "Cfg.Is Child?"=w584:bool)
        n260 = call "Pololu.Mgr - Disconnect.vi"("PololuCtrl in"=w591) -> ("PololuCtrl out"=w590:refnum<class "PololuCtrl.lvclass">)  [unwired: 9 in, 1 out]
        n261 = Not(x=w584) -> (.not. x?=w582:bool)
        n262 = And(x=w583, y=w582) -> (x .and. y?=w581:bool)
        n263 = call "Pololu.Mgr - Save Config.vi"("PololuCtrl in"=w590) -> ("error out"=w587:errorcluster)  [unwired: 9 in, 1 out]
        n264 = invoke on="Connected" class="Bool (strict)" method="Reinit To Default"() -> ()  [unwired: 3 in, 3 out]
        n265 = flat-sequence {
          tunnel: [w594] -> w585
          tunnel: w586 -> [w594]
          frame #0 {
            n266 = call <vilib>:"Event Log.Debug Util, Print to File.vi"("Enable"=FALSE, "Message"="App Exit") -> ()  [unwired: 10 in]
          }
        }
        n267 = call <vilib>:"Module.Destructor.vi"("error in"=w587, "Sys"=w588) -> ("error out"=w586:errorcluster)  [unwired: 9 in]
        n268 = case shown="True" w581 {
          tunnel: w585 -> [_ _]
          frame False {
          }
          frame True {
            n269 = Quit LabVIEW() -> ()  [unwired: 1 in]
          }
        }
      }
    }
  }
  n270 = while {
    tunnel: w3 -> [w598]
    tunnel: w3 -> [w596]
    stop <- w600 stop-if-true
    n271 = Unbundle By Name(w598) -> ("Stop.Ref"=w597:refnum<event-registration>, "Main Q"=w599:refnum<queue>)
    n272 = event shown="[0] \"Disconnect\", \"Connect\": Value Change" {
      selector: w597 -> [_ _ _ _ _ _ _ _ _ _ _ _ _ _ _ _ _]
      dyn-events: _ -> [_ _ _ _ _ _ _ _ _ _ _ _ _ _ _ _ _]
      timeout: _ -> [_ _ _ _ _ _ _ _ _ _ _ _ _ _ _ _ _]
      tunnel: w599 -> [w605 w607 w609 w610 w613 w617 w631 w638 w657 w671 w673 w686 _ w702 w717 w719 _]
      tunnel: [_ _ _ _ _ _ _ _ _ _ _ _ _ _ _ w722 TRUE] -> w600
      tunnel: w596 -> [_ _ _ _ _ _ _ _ _ _ _ _ _ _ _ w720 _]
      event "Disconnect", "Connect": Value Change {
        n273 = event-data() -> ()  [unwired: 1 in, 6 out]
        n274 = Select(t="Connect", s="Connect", f="Disconnect") -> (s? t:f=w602:string)
        n275 = call <vilib>:"Q.Enqueue Task.vi"("Task Name"=w602, "Q In"=w605) -> ()  [unwired: 8 in, 2 out]
      }
      event "Set Speed": Value Change {
        n276 = event-data() -> ()  [unwired: 1 in, 6 out]
        n277 = call <vilib>:"Q.Enqueue Task.vi"("Task Name"="Set Speed", "Q In"=w607) -> ()  [unwired: 8 in, 2 out]
      }
      event "Set Accel": Value Change {
        n278 = event-data() -> ()  [unwired: 1 in, 6 out]
        n279 = call <vilib>:"Q.Enqueue Task.vi"("Task Name"="Set Accel", "Q In"=w609) -> ()  [unwired: 8 in, 2 out]
      }
      event "Get Pos": Value Change {
        n280 = event-data() -> ()  [unwired: 1 in, 6 out]
        n281 = call <vilib>:"Q.Enqueue Task.vi"("Task Name"="Get Status", "Q In"=w610) -> ()  [unwired: 8 in, 2 out]
      }
      event "Get Errors": Value Change {
        n282 = event-data() -> ()  [unwired: 1 in, 6 out]
        n283 = call <vilib>:"Q.Enqueue Task.vi"("Task Name"="Read Errors", "Q In"=w613) -> ()  [unwired: 8 in, 2 out]
      }
      event "Left Cmd Pos (Deg)": Value Change {
        w615 = "Get Status"
        w618 = "Set Left Pos"
        n284 = event-data() -> ()  [unwired: 1 in, 6 out]
        n285 = call <vilib>:"Scheduler.AddTask.vi"("Interval(s)"=0.2, "Task Name"=w618, "Sched Name"=w618, "Q In"=w617) -> ("Q Out"=w616:refnum<queue>)  [unwired: 6 in, 1 out]
        n286 = call <vilib>:"Scheduler.AddTask.vi"("Interval(s)"=0.3, "Task Name"=w615, "Sched Name"=w615, "Q In"=w616) -> ()  [unwired: 6 in, 2 out]
      }
      event "L Step Up", "L Step Dwn", "R Step Up", "R Step Dwn": Value Change {
        n287 = event-data() -> ()  [unwired: 1 in, 6 out]
        n288 = Or(x="L Step Up", y="L Step Dwn") -> (x .or. y?=w625:bool)
        n289 = Or(x="L Step Up", y="R Step Up") -> (x .or. y?=w622:bool)
        n290 = call <vilib>:"Q.Enqueue Task.vi"("Task Name"="Set Left Pos", "Q In"=w631) -> ("Q Out"=w629:refnum<queue>)  [unwired: 8 in, 1 out]
        n291 = Select(t=1.0, s=w622, f=-1.0) -> (s? t:f=w621:dbl)
        n292 = call <vilib>:"Q.Enqueue Task.vi"("Task Name"="Get Status", "Q In"=w629) -> ()  [unwired: 8 in, 2 out]
        n293 = case shown="False" w625 {
          tunnel: w621 -> [w632 w635]
          frame False {
            n294 = local read "Right Cmd Pos (Deg)"() -> (w634:dbl)
            n295 = Add(x=w634, y=w632) -> (x+y=w633:dbl)
            n296 = local write "Right Cmd Pos (Deg)"(w633) -> ()
          }
          frame True {
            n297 = local read "Left Cmd Pos (Deg)"() -> (w637:dbl)
            n298 = Add(x=w637, y=w635) -> (x+y=w636:dbl)
            n299 = local write "Left Cmd Pos (Deg)"(w636) -> ()
          }
        }
      }
      event "Right Cmd Pos (Deg)": Value Change {
        w640 = "Get Status"
        w642 = "Set Right Pos"
        n300 = event-data() -> ()  [unwired: 1 in, 6 out]
        n301 = call <vilib>:"Scheduler.AddTask.vi"("Interval(s)"=0.2, "Task Name"=w642, "Sched Name"=w642, "Q In"=w638) -> ("Q Out"=w641:refnum<queue>)  [unwired: 6 in, 1 out]
        n302 = call <vilib>:"Scheduler.AddTask.vi"("Interval(s)"=0.3, "Task Name"=w640, "Sched Name"=w640, "Q In"=w641) -> ()  [unwired: 6 in, 2 out]
      }
      event "L Go To Pos 1", "L Go To Pos 0", "R Go To Pos 1", "R Go To Pos 0": Value Change {
        n303 = event-data() -> ()  [unwired: 1 in, 6 out]
        n304 = Select(t=T8."Right Pos 0", s="R Go To Pos 0", f=T8."Right Pos 1") -> (s? t:f=w648:T8)
        n305 = Select(t=T8."Left Pos 1", s="L Go To Pos 1", f=w648) -> (s? t:f=w651:T8)
        n306 = Select(t=T8."Left Pos 0", s="L Go To Pos 0", f=w651) -> (s? t:f=w653:T8)
        n307 = To Variant(anything=w653) -> (Variant=w647:variant)
        n308 = call <vilib>:"Q.Enqueue Task.vi"("Data1"=w647, "Task Name"="Go To Saved Pos", "Q In"=w657) -> ("Q Out"=w655:refnum<queue>)  [unwired: 7 in, 1 out]
        n309 = call <vilib>:"Q.Enqueue Task.vi"("Task Name"="Get Status", "Q In"=w655) -> ()  [unwired: 8 in, 2 out]
      }
      event "L Set Upper Stop", "R Set Upper Stop", "L Set Lower Stop", "R Set Lower Stop": Value Change {
        n310 = event-data() -> ()  [unwired: 1 in, 6 out]
        n311 = Select(t=T8."Right Upper Stop", s="R Set Upper Stop", f=T8."Right Lower Stop") -> (s? t:f=w659:T8)
        n312 = Select(t=T8."Left Lower Stop", s="L Set Lower Stop", f=w659) -> (s? t:f=w664:T8)
        n313 = Select(t=T8."Left Upper Stop", s="L Set Upper Stop", f=w664) -> (s? t:f=w667:T8)
        n314 = To Variant(anything=w667) -> (Variant=w668:variant)
        n315 = call <vilib>:"Q.Enqueue Task.vi"("Data1"=w668, "Task Name"="Store Stop Position", "Q In"=w671) -> ()  [unwired: 7 in, 2 out]
      }
      event "Reset Stops": Value Change {
        n316 = event-data() -> ()  [unwired: 1 in, 6 out]
        n317 = call <vilib>:"Q.Enqueue Task.vi"("Task Name"="Reset Stop Positions", "Q In"=w673) -> ()  [unwired: 8 in, 2 out]
      }
      event "L Set Pos 1", "L Set Pos 0", "R Set Pos 1", "R Set Pos 0": Value Change {
        n318 = event-data() -> ()  [unwired: 1 in, 6 out]
        n319 = Select(t=T8."Right Pos 0", s="R Set Pos 0", f=T8."Right Pos 1") -> (s? t:f=w677:T8)
        n320 = Select(t=T8."Left Pos 1", s="L Set Pos 1", f=w677) -> (s? t:f=w680:T8)
        n321 = Select(t=T8."Left Pos 0", s="L Set Pos 0", f=w680) -> (s? t:f=w682:T8)
        n322 = To Variant(anything=w682) -> (Variant=w683:variant)
        n323 = call <vilib>:"Q.Enqueue Task.vi"("Data1"=w683, "Task Name"="Store Position", "Q In"=w686) -> ()  [unwired: 7 in, 2 out]
      }
      event "Pos0 Invert", "Pos1 Invert": Value Change {
        n324 = event-data() -> ()  [unwired: 1 in, 6 out]
        n325 = local read "Pos1 Invert"() -> (w687:bool)
        n326 = local read "Pos0 Invert"() -> (w688:bool)
        n327 = property on="Left Cmd Pos (Deg)" class="Slide (strict)"("Scale.Flipped"=w688) -> ()  [unwired: 2 in, 2 out]
        n328 = property on="Right Cmd Pos (Deg)" class="Slide (strict)"("Scale.Flipped"=w687) -> ()  [unwired: 2 in, 2 out]
      }
      event "Move Funct": Value Change {
        # "Move(PositionID,[Devices, WaitTtillDone,TimeOut])"
        n329 = event-data() -> ()  [unwired: 1 in, 6 out]
        n330 = Format Into String("Mov Device") -> (resulting string=w696:string)  [unwired: 3 in, 1 out]
        n331 = Number To Decimal String(number="Mov PosID") -> (decimal integer string=w698:string)  [unwired: 1 in]
        n332 = Select(t="1", s="WaitTillDone", f="0") -> (s? t:f=w692:string)
        n333 = Number To Fractional String(number="Mov Timeout") -> (F-format string=w690:string)  [unwired: 3 in]
        n334 = Build Array(w698, w696, w692, w690) -> (w699:string[])
        n335 = To Variant(anything=w699) -> (Variant=w703:variant)
        n336 = call <vilib>:"Q.Enqueue Function.vi"("RetSubCmd"="Local RTN", "Data1"=w703, "Task Name"="Move", "Q In"=w702) -> ()  [unwired: 5 in, 3 out]
      }
      event "Move All to 1", "Move All to 0", "Move All to 3": Value Change {
        # "Move(PositionID,[Devices, WaitTtillDone,TimeOut])"
        n337 = event-data() -> ()  [unwired: 1 in, 6 out]
        n338 = Select(t="0", s="Move All to 0", f="3") -> (s? t:f=w707:string)
        n339 = Select(t="1", s="Move All to 1", f=w707) -> (s? t:f=w713:string)
        n340 = Build Array(w713, "All", "False", "1") -> (w715:string[])
        n341 = To Variant(anything=w715) -> (Variant=w718:variant)
        n342 = call <vilib>:"Q.Enqueue Function.vi"("RetSubCmd"="Local RTN", "Data1"=w718, "Task Name"="Move", "Q In"=w717) -> ()  [unwired: 5 in, 3 out]
      }
      event Panel Close? {
        n343 = event-data() -> ()  [unwired: 1 in, 4 out]
        n344 = Unbundle By Name(w720) -> ("Cfg.Is Child?"=w721:bool)
        n345 = case shown="True" w721 {
          tunnel: w719 -> [w726 w729]
          tunnel: [TRUE TRUE] -> w723
          tunnel: [TRUE FALSE] -> w722
          tunnel: [_ w727] -> _
          frame False {
            # "Parent - Exit"
            n346 = call <vilib>:"Q.Enqueue Exit.vi"("Q In"=w726) -> ()  [unwired: 9 in, 2 out]
          }
          frame True {
            # "Child - Hide Panel and if was \nin a subpanel, return to subpanel."
            n347 = call <vilib>:"Module.Window, Q Task.vi"("Action"=Window.Task,_Action."Return to SubPanel()", "Q In"=w729) -> ("error out"=w727:errorcluster)  [unwired: 8 in, 1 out]
          }
        }
        n348 = event-data("Discard?"=w723) -> ()  [unwired: 1 in, 1 out]
      }
      event User Event {
        n349 = event-data() -> ()  [unwired: 1 in, 5 out]
      }
    }
  }
